vi "Array Parser.vi"() -> (1 "Auto Routines":string[](array[string]), 2 "List of Files":string[](array[string]), 3 "CSV Data":string[][][](array[string]))   [LabVIEW 2015]
uses:
  <vilib>/Utility/sysdir.llb/System Directory Type.ctl
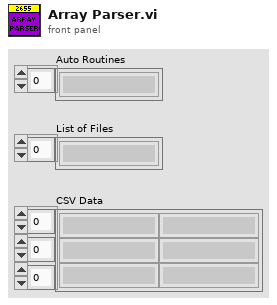
[diagram p1: front panel]
types:
  T1 = typedef "System Directory Type.ctl" = i32
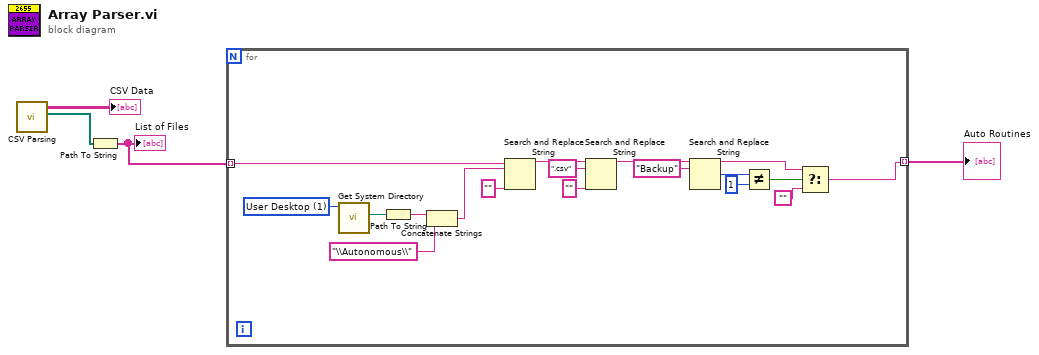
[diagram p0: block diagram]
diagram:
  n1 = call "CSV Parsing.vi"() -> ("Files in Directory"=w3:path[], "CSV Data"=→"CSV Data":string[][][])  [unwired: 10 in]
  n2 = Path To String(path=w3) -> (string=w2:string[])
  "List of Files" <- w2
  n3 = for {
    tunnel: w2 -> [w13] mode=indexing
    tunnel: [w6] -> w1 mode=indexing
    w18 = T1 1 items=["User Home"=0, "User Desktop"=1, "User Documents"=2, "User Application Data"=3, "User Preferences"=4, "User Temporary"=5, "Public Documents"=6, "Public Application Data"=7, "Public Preferences"=8, "Public Cache"=13, "System Core Libraries"=9, "System Installed Libraries"=10, "Application Files"=11, "Boot Volume Root"=12] ("system directory type")
    n4 = call <vilib>:"Get System Directory.vi"("system directory type"=w18) -> ("system directory"=w17:path)  [unwired: 10 in]
    n5 = Path To String(path=w17) -> (string=w16:string)
    n6 = Concatenate Strings(w16, "\\Autonomous\\" ("string")) -> (w14:string)
    n7 = Search and Replace String(input string=w13, search string=w14, replace string="" ("replace string (\"\")")) -> (result string=w19:string)  [unwired: 5 in, 3 out]
    n8 = Search and Replace String(input string=w19, search string=".csv", replace string="" ("replace string (\"\")")) -> (result string=w11:string)  [unwired: 5 in, 3 out]
    n9 = Search and Replace String(input string=w11, search string="Backup") -> (result string=w7:string, number of replacements=w8:i32)  [unwired: 6 in, 2 out]
    n10 = Not Equal?(x=w8, y=1) -> (x != y?=w9:bool)
    n11 = Select(t=w7, s=w9, f="") -> (s? t:f=w6:string)
  }
  "Auto Routines" <- w1
